vi "Configure Marker Function.vi"(7 "Marker Function":T1, 8 "error in (no error)":errorcluster, 10 "Marker Number (1)":u32=1 min=1, 11 "SA-ESA in":refnum<class "SA-ESA.lvclass">) -> (0 "error out":errorcluster, 3 "SA-ESA out":refnum<class "SA-ESA.lvclass">)   [LabVIEW 2020, in "SA-ESA.lvclass"]
uses:
  SA-ESA.lvclass
  C:/Sandbox/Git_Sandbox/WiSpry Test Framework source code (LV20)/WiSpry Test Framework/Instruments/Instrument.lvclass
  Controls/Marker Functions.ctl
  Instrument.lvclass/Instrument.ctl
  Instrument.lvclass
  Spectrum Analyzer.lvclass
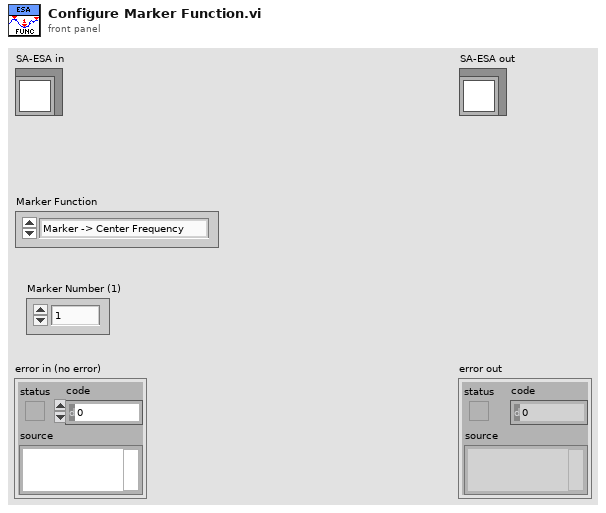
[diagram p1: front panel]
types:
  T1 = typedef "Spectrum Analyzer.lvclass/Marker Functions.ctl" = enum16{"Marker -> Center Frequency", "Marker -> Reference Level"}
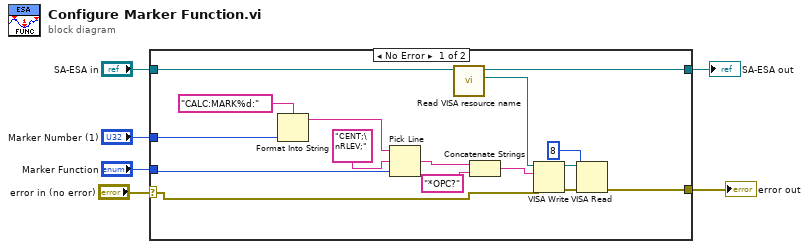
[diagram p0: block diagram]
diagram:
  n1 = case shown="No Error" "error in (no error)" {
    selector: "error in (no error)" -> [w8 w23]
    tunnel: "SA-ESA in" -> [w15 w24]
    tunnel: "Marker Number (1)" -> [w21 _]
    tunnel: "Marker Function" -> [w20 _]
    tunnel: [w13 w24] -> w2
    tunnel: [w7 w23] -> w1
    frame No Error {
      n2 = Format Into String(format string="CALC:MARK%d:", w21) -> (resulting string=w19:string)  [unwired: 2 in, 1 out]
      n3 = Pick Line(string ("")=w19, multi-line string="CENT;\nRLEV;", line index=w20) -> (output string=w17:string)
      n4 = call "Read VISA resource name.vi"("Instrument in"=w15) -> ("VISA resource name"=w14:refnum<visa-resource-name>, "Instrument out"=w13:refnum<class "SA-ESA.lvclass">)  [unwired: 9 in]
      n5 = Concatenate Strings(w17, "*OPC?" ("string")) -> (w12:string)
      n6 = VISA Write(VISA resource name=w14, write buffer=w12, error in (no error)=w8) -> (VISA resource name out=w11:refnum<visa-resource-name>, error out=w9:errorcluster)  [unwired: 1 out]
      n7 = VISA Read(VISA resource name=w11, byte count=u32 8, error in (no error)=w9) -> (error out=w7:errorcluster)  [unwired: 3 out]
    }
    frame Error {
    }
  }
  "error out" <- w1
  "SA-ESA out" <- w2
